vi "pf_Set_Camera_Property_Int.vi"(8 "error in (no error)":errorcluster, 9 "Property Value":u32, 10 "Property Name":string, 11 "IMAQ Session in":refnum<k11>) -> (0 "error out":errorcluster, 2 "Property Name out":string, 3 "IMAQ Session out":refnum<k11>)   [LabVIEW 2025, in "Photonfocus_Toolkit.lvlib"]
doc: "Sets the value of a Integer type property."
uses:
  Photonfocus_Toolkit.lvlib
  _Private/Controls/pf_Camera_ctrl_mngr_action.ctl
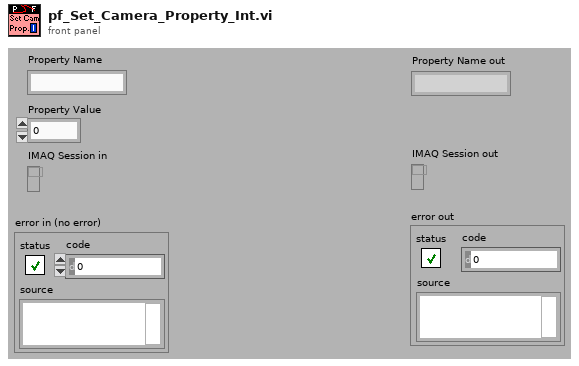
[diagram p1: front panel]
types:
  T1 = typedef "Photonfocus_Toolkit.lvlib/pf_Camera_ctrl_mngr_action.ctl" = enum16{"Create", "Destroy", "Set", "Get"}
  T2 = typedef "Photonfocus_Toolkit.lvlib/pf_Camera_Control.ctl" = cluster{"Port Name":string, "Port Number":i32, "IMAQ Session":refnum<k11>, "PeakDetector_Mode":T3, "Window.W":u32, "Window.H":u32}
  T3 = typedef "Photonfocus_Toolkit.lvlib/pf_PeakDetector_Mode.ctl" = enum16{"Undefined", "2D only", "2D and 3D", "3D only"}
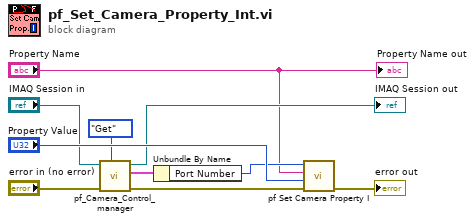
[diagram p0: block diagram]
diagram:
  n1 = call "pf_Camera_Control_manager.vi"("Action"=pf_Camera_ctrl_mngr_action."Get", "error in (no error)"="error in (no error)", "IMAQ Session in"="IMAQ Session in") -> ("error out"=w7:errorcluster, "Camera Control out"=w3:T2, "IMAQ Session out"=→"IMAQ Session out":refnum<k11>)  [unwired: 1 in, 5 out]
  n2 = Unbundle By Name(w3) -> ("Port Number"=w2:i32)
  n3 = call "pf Set Camera Property I.vi"("error in (no error)"=w7, "iValue"="Property Value", "pProperty"="Property Name", "iPort"=w2) -> ("error out"=→"error out":errorcluster)  [unwired: 7 out]
  "Property Name out" <- "Property Name"
